vi "TB-Save SPL History.vi"(0 "state":T4, 1 "Log in":T2, 5 "XYGraph in":refnum<vi>, 7 "date/time string":string, 9 "history":cluster{dbl[], dbl[]}[](array[cluster]), 12 "Exposure parameters":T1={"Low cutoff (kHz)"=8.0, "High cutoff (kHz)"=16.0, "Duration (min)"=120.0, "dB SPL"=100.0, "Waveform"=enum."Noise", "WAVfile"=path "", "refWav"=path "", "use mic correction"=FALSE, "micCorrFile"=path "", "Pistonphone Level (dB SPL)"=0.0, "Sampling rate (Hz)"=0.0, "Buffer length (s)"=0.0, "Stream mic"=FALSE, "Fine adjust"={"Max"=0.0, "Min"=0.0}, "Mic gain"=0.0, "atten"=0.0, "resol (Hz)"=0.0, "navgs"=0, "Allow Slack"=FALSE, "max starts"=0, "Freq (kHz)"=8.0, "Tma (s)"=0.0, "Streamed"=[], "Drive"="", "Speaker"="", "Mic"=""}) -> (15 "error out":errorcluster)   [LabVIEW 2020]
uses:
  Typedefs/TB-Runtime state.ctl
  <vilib>/sound2/lvsound2.llb/Sound File Refnum.ctl
  Typedefs/TB-Setup Log.ctl
  Typedefs/TB-Log.ctl
  Typedefs/TB-Slack State.ctl
  Typedefs/TB-Parameters.ctl
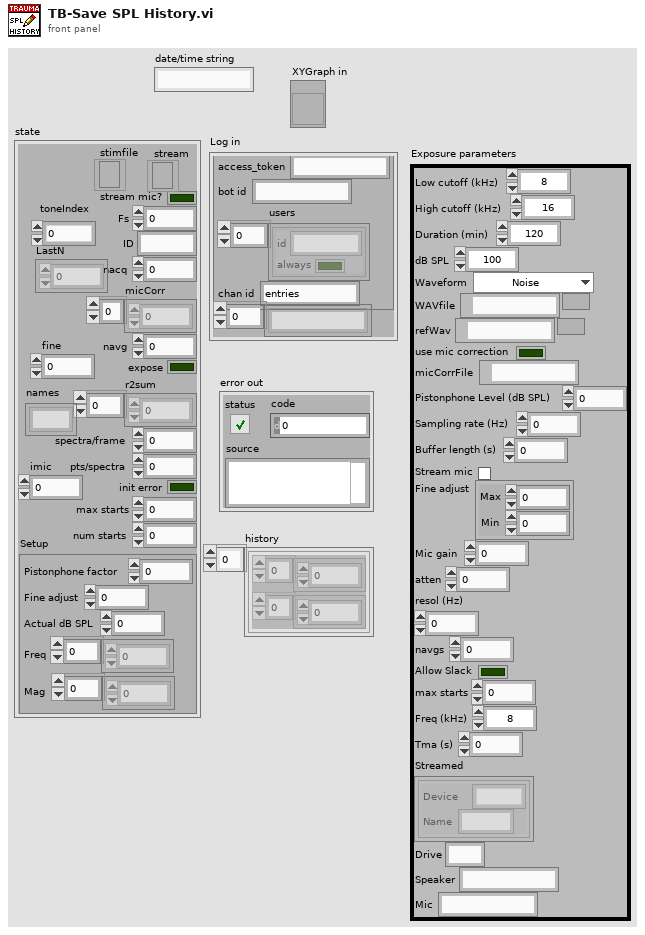
[diagram p1: front panel]
types:
  T1 = typedef "TB-Parameters.ctl" = cluster{"Low cutoff (kHz)":dbl, "High cutoff (kHz)":dbl, "Duration (min)":dbl, "dB SPL":dbl, "Waveform":enum16{"Noise", "File", "Tone"}, "WAVfile":path, "refWav":path, "use mic correction":bool, "micCorrFile":path, "Pistonphone Level (dB SPL)":dbl, "Sampling rate (Hz)":dbl, "Buffer length (s)":dbl, "Stream mic":bool, "Fine adjust":cluster{"Max":dbl, "Min":dbl}, "Mic gain":dbl, "atten":dbl, "resol (Hz)":dbl, "navgs":i32, "Allow Slack":bool, "max starts":i32, "Freq (kHz)":dbl, "Tma (s)":dbl, "Streamed":cluster{"Device":string, "Name":string}[], "Drive":string, "Speaker":string, "Mic":string}
  T2 = typedef "TB-Log.ctl" = cluster{"Slack":T3, "entries":string[]}
  T3 = typedef "TB-Slack State.ctl" = cluster{"access_token":string, "bot id":string, "users":cluster{"id":string, "always":bool}[], "chan id":string}
  T4 = typedef "TB-Runtime state.ctl" = cluster{"stimfile":T5, "stream mic?":bool, "Fs":dbl, "ID":string, "micCorr":dbl[], "navg":i32, "r2sum":dbl[], "expose":bool, "spectra/frame":i32, "pts/spectra":i32, "nacq":i32, "init error":bool, "max starts":i32, "num starts":i32, "Setup":T6, "toneIndex":i32, "LastN":dbl[], "fine":dbl, "imic":i32, "stream":refnum<file>, "names":string[]}
  T5 = typedef "Sound File Refnum.ctl" = refnum<file>
  T6 = typedef "TB-Setup Log.ctl" = cluster{"Pistonphone factor":dbl, "Fine adjust":dbl, "Actual dB SPL":dbl, "Freq":dbl[], "Mag":dbl[]}
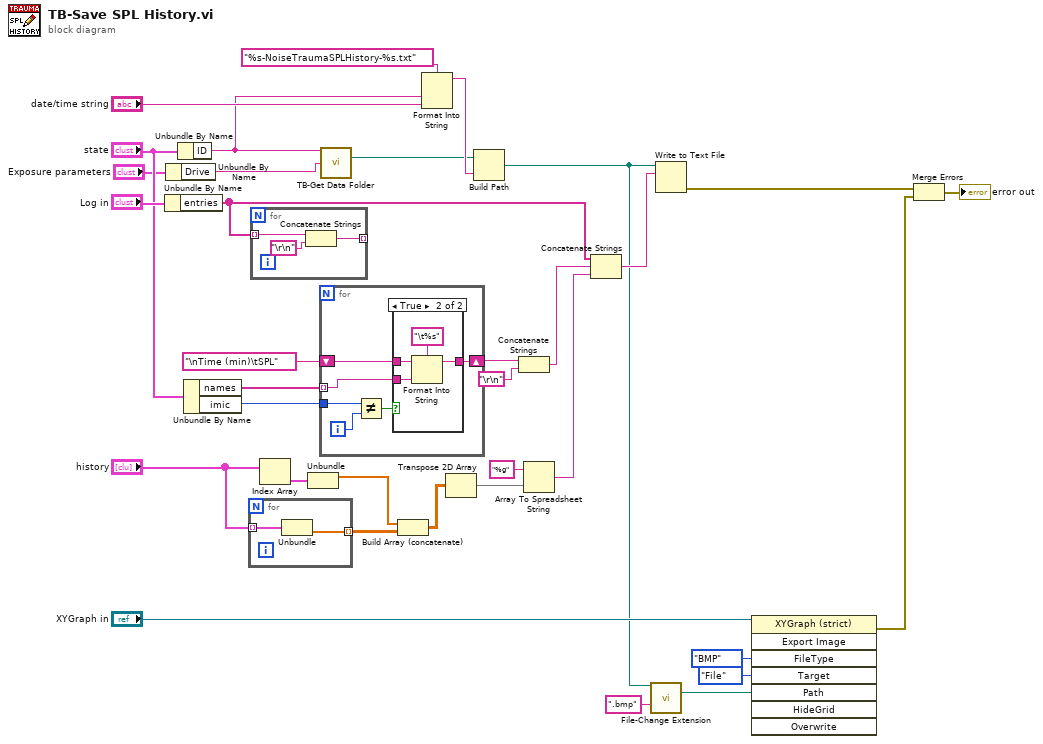
[diagram p0: block diagram]
diagram:
  n1 = Unbundle By Name("Log in") -> ("entries"=w23:string[])
  n2 = Unbundle By Name("Exposure parameters") -> ("Drive"=w2:string)
  n3 = Unbundle By Name("state") -> ("ID"=w1:string)
  n4 = Unbundle By Name("state") -> ("names"=w5:string[], "imic"=w4:i32)
  n5 = for {
    tunnel: "history" -> [w36] mode=indexing
    tunnel: [w35] -> w32 mode=indexing
    n6 = Unbundle(w36) -> (w35:dbl[])  [unwired: 1 out]
  }
  n7 = for {
    tunnel: w23 -> [w39] mode=indexing
    tunnel: [w37] -> _ mode=indexing
    n8 = Concatenate Strings(w39, "\r\n") -> (w37:string)
  }
  n9 = Index Array(array="history") -> (element=w12:cluster{dbl[], dbl[]})  [unwired: 1 in]
  n10 = Unbundle(w12) -> (w11:dbl[])  [unwired: 1 out]
  n11 = for {
    shift-right: [w44] -> w8
    shift-left: "\nTime (min)\tSPL" ("string") -> [w45]
    tunnel: w5 -> [w43] mode=indexing
    tunnel: w4 -> [w42]
    i -> [w41]
    n12 = Not Equal?(x=w42, y=w41) -> (x != y?=w40:bool)
    n13 = case shown="True" w40 {
      tunnel: w45 -> [w46 w50]
      tunnel: [w46 w49] -> w44
      tunnel: w43 -> [_ w48]
      frame False {
      }
      frame True {
        n14 = Format Into String(format string="\t%s", initial string=w50, w48) -> (resulting string=w49:string)  [unwired: 1 in, 1 out]
      }
    }
  }
  n15 = call "TB-Get Data Folder.vi"("ID"=w1, "Drive"=w2) -> ("Data folder"=w25:path)  [unwired: 12 in, 1 out]
  n16 = Build Array (concatenate)(w11, w32) -> (w31:dbl[][])
  n17 = Format Into String(format string="%s-NoiseTraumaSPLHistory-%s.txt", w1, "date/time string") -> (resulting string=w33:string)  [unwired: 2 in, 1 out]
  n18 = Transpose 2D Array(2D array=w31) -> (transposed array=w30:dbl[][])
  n19 = Build Path(base path=w25, name or relative path=w33) -> (appended path=w19:path)
  n20 = Concatenate Strings(w8, "\r\n") -> (w7:string)
  n21 = Array To Spreadsheet String(array=w30, 3:"%g" ("format string")) -> (spreadsheet string=w28:string)  [unwired: 1 in]
  n22 = Concatenate Strings(w23, w7, w28) -> (w27:string)
  n23 = call "File-Change Extension.vi"("Path"=w19, "new extension"=".bmp") -> ("new path"=w18:path)  [unwired: 12 in, 1 out]
  n24 = Write to Text File(file (use dialog)=w19, text=w27) -> (error out=w26:errorcluster)  [unwired: 2 in, 2 out]
  n25 = invoke class="XYGraph (strict)" method="Export Image"(reference="XYGraph in", "FileType"=enum32{"BMP", "EPS", "EMF", "PICT"}."BMP" ("File Type"), "Target"=enum32{"File", "Clipboard"}."File", "Path"=w18) -> (error out=w14:errorcluster)  [unwired: 4 in, 7 out]
  n26 = Merge Errors(w26, w14) -> (→"error out":errorcluster)
